vi "Results-FGV.vi"(8 "error in":errorcluster, 9 "Mode":enum16{"Write", "Read", "Delete"}(ring), 10 "Encoder-data":T1(array[cluster]), 11 "Analog-data":sgl[][](array[numeric])) -> (0 "error out":errorcluster, 2 "Encoder-data out":T1(array[cluster]), 3 "Analog-data out":sgl[][](array[numeric]))   [LabVIEW 2016]
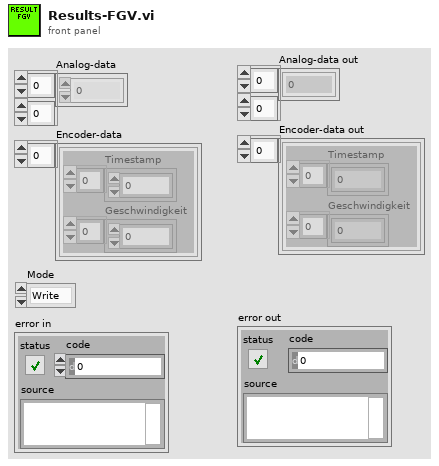
[diagram p1: front panel]
types:
  T1 = cluster{"Timestamp":sgl[], "Geschwindigkeit":sgl[]}[]
  T2 = cluster{"Timestamp":sgl[], "Geschwindigkeit":sgl[]}
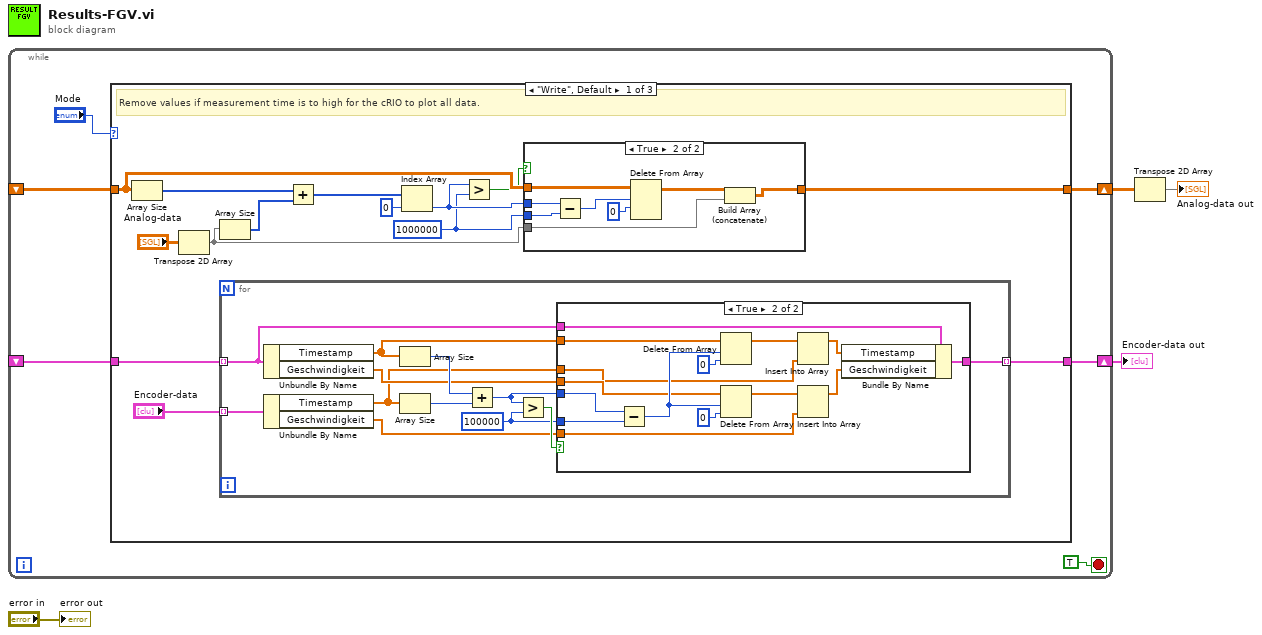
[diagram p0: block diagram]
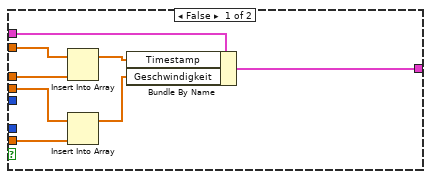
[diagram p2: hidden frame]
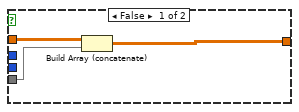
[diagram p3: hidden frame]
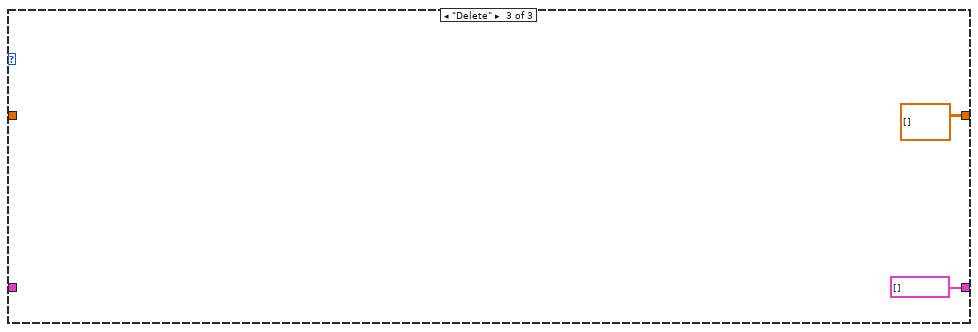
[diagram p5: hidden frame]
diagram:
  n1 = while {
    shift-right: [w8] -> w3
    shift-left: _ -> [w7]
    shift-right: [w6] -> w2
    shift-left: _ -> [w5]
    stop <- TRUE stop-if-true
    n2 = case shown="\"Write\", Default" "Mode" {
      tunnel: [w16 w72 sgl[][] []] -> w8
      tunnel: w7 -> [w21 w72 _]
      tunnel: [w13 w71 T1 [] ("Encoder-data")] -> w6
      tunnel: w5 -> [w15 w71 _]
      frame "Write", Default {
        w18 = 1000000 ("y")
        # "Remove values if measurement time is to high for the cRIO to plot all data."
        n3 = Array Size(array=w21) -> (size(s)=w24:i32[])
        n4 = Transpose 2D Array(2D array="Analog-data") -> (transposed array=w11:sgl[][])
        n5 = Array Size(array=w11) -> (size(s)=w23:i32[])
        n6 = for {
          tunnel: w15 -> [w26] mode=indexing
          tunnel: "Encoder-data" -> [w36] mode=indexing
          tunnel: [w25] -> w13 mode=indexing
          w31 = 100000 ("y")
          n7 = Unbundle By Name(w26) -> ("Timestamp"=w30:sgl[], "Geschwindigkeit"=w29:sgl[])
          n8 = Unbundle By Name(w36) -> ("Timestamp"=w28:sgl[], "Geschwindigkeit"=w27:sgl[])
          n9 = Array Size(array=w30) -> (size(s)=w35:i32)
          n10 = Array Size(array=w28) -> (size(s)=w34:i32)
          n11 = Add(x=w35, y=w34) -> (x+y=w32:i32)
          n12 = Greater?(x=w32, y=w31) -> (0:w33:bool)
          n13 = case shown="True" w33 {
            tunnel: w32 -> [_ w59]
            tunnel: w31 -> [_ w58]
            tunnel: w30 -> [w43 w57]
            tunnel: w29 -> [w38 w53]
            tunnel: w28 -> [w42 w51]
            tunnel: w27 -> [w37 w49]
            tunnel: w26 -> [w44 w48]
            tunnel: [w40 w45] -> w25
            frame False {
              n14 = Insert Into Array(array=w43, new element=w42) -> (w41:sgl[])  [unwired: 1 in]
              n15 = Insert Into Array(array=w38, new element=w37) -> (w39:sgl[])  [unwired: 1 in]
              n16 = Bundle By Name(cluster=w44, "Timestamp"=w41, "Geschwindigkeit"=w39) -> (w40:T2)
            }
            frame True {
              n17 = Subtract(x=w59, y=w58) -> (x-y=w54:i32)
              n18 = Delete From Array(array=w57, length=w54, index=0) -> (array with subset deleted=w52:sgl[])  [unwired: 1 out]
              n19 = Delete From Array(array=w53, length=w54, index=0) -> (array with subset deleted=w50:sgl[])  [unwired: 1 out]
              n20 = Insert Into Array(array=w52, new element=w51) -> (w47:sgl[])  [unwired: 1 in]
              n21 = Insert Into Array(array=w50, new element=w49) -> (w46:sgl[])  [unwired: 1 in]
              n22 = Bundle By Name(cluster=w48, "Timestamp"=w47, "Geschwindigkeit"=w46) -> (w45:T2)
            }
          }
        }
        n23 = Add(x=w24, y=w23) -> (x+y=w22:i32[])
        n24 = Index Array(array=w22, index=0) -> (element=w19:i32)
        n25 = Greater?(x=w19, y=w18) -> (0:w20:bool)
        n26 = case shown="True" w20 {
          tunnel: w21 -> [w62 w70]
          tunnel: w19 -> [_ w69]
          tunnel: w18 -> [_ w68]
          tunnel: w11 -> [w61 w64]
          tunnel: [w60 w63] -> w16
          frame False {
            n27 = Build Array (concatenate)(w62, w61) -> (w60:sgl[][])
          }
          frame True {
            n28 = Subtract(x=w69, y=w68) -> (x-y=w67:i32)
            n29 = Delete From Array(array=w70, length=w67, index (row)=0) -> (array with subset deleted=w65:sgl[][])  [unwired: 1 in, 1 out]
            n30 = Build Array (concatenate)(w65, w64) -> (w63:sgl[][])
          }
        }
      }
      frame "Read" {
      }
      frame "Delete" {
      }
    }
  }
  "Encoder-data out" <- w2
  n31 = Transpose 2D Array(2D array=w3) -> (transposed array=→"Analog-data out":sgl[][])
  "error out" <- "error in"
